vi "fearConditioningOld.vi"() -> ()   [LabVIEW 2010]
uses:
  <vilib>/DAQmx/write.llb/DAQmx Write (Digital Bool 1Line 1Point).vi
  GlobalFear.vi
  <vilib>/daqmx/miscellaneous.llb/DAQmx Fill In Error Info.vi
  <vilib>/measure/NI_MABase.lvlib
panel:
  in  "Pre CS\ntime":dbl=50.0
  in  "stop 2":bool
  in  "stop":bool
  out "Start":bool
  in  "Start":bool
  out "Copleted":bool
  in  "Frequency":dbl=10000.0
  out "Started":bool
  out "Counter":dbl
  in  "ITI":dbl=180.0
  in  "# repeats":dbl=10.0
  out "Shock":bool
  out "Elapsed  Time":dbl format="%#_3g"
  in  "Shock\nDelay":dbl=-1.0
  in  "Shock \nDuration":dbl=-1.0
  in  "Audio \nDuration":dbl=30.0
  out "Audio":bool
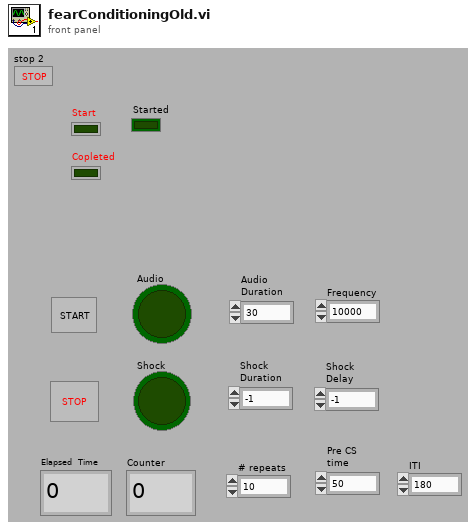
[diagram p1: front panel]
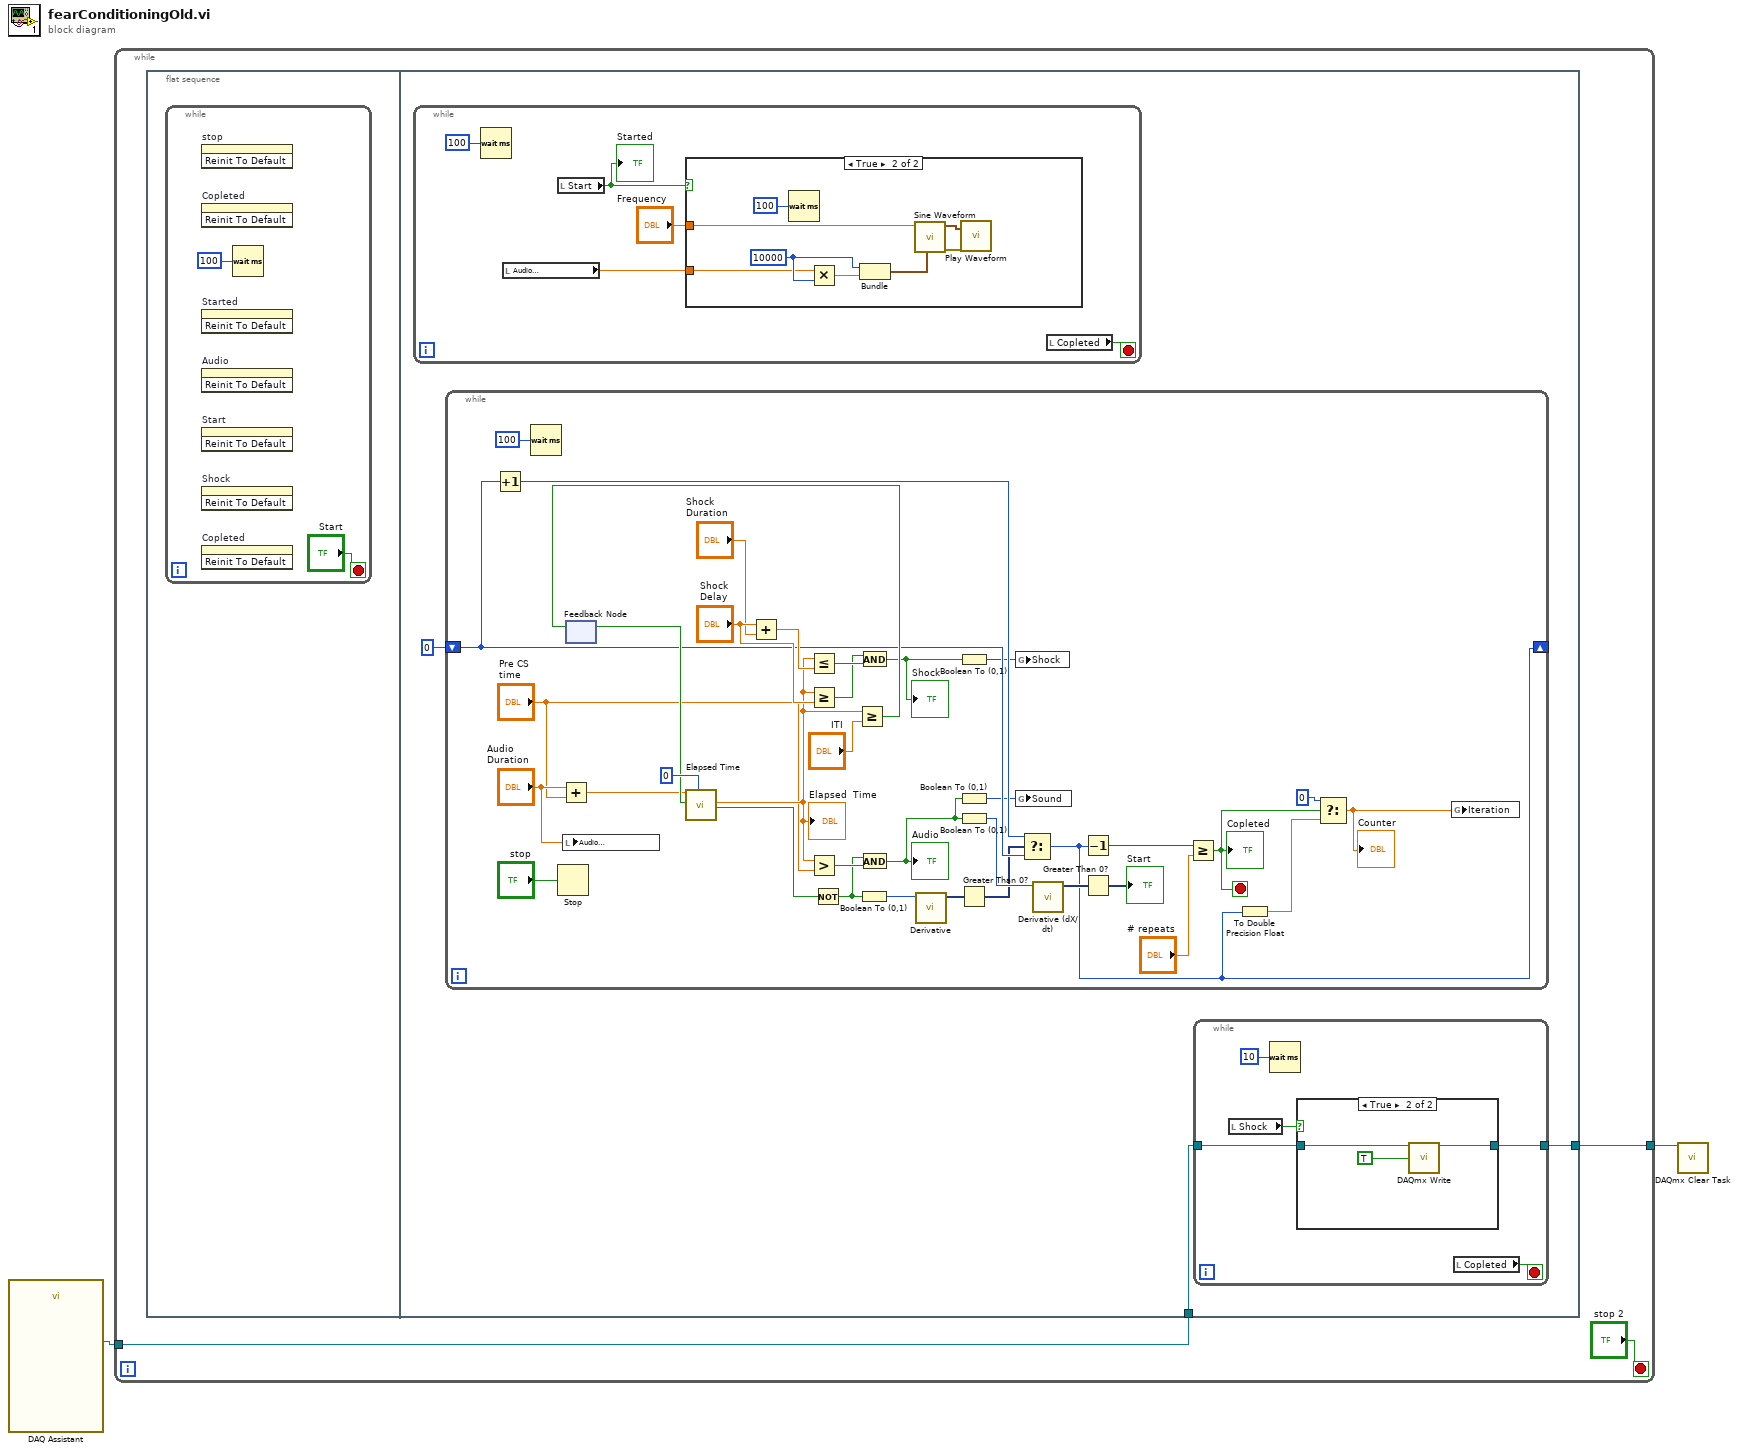
[diagram p0: block diagram]
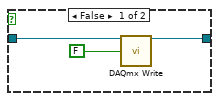
[diagram p2: hidden frame]
diagram:
  n1 = call "DAQ Assistant"() -> ("task out"=w2:refnum<k21>)  [unwired: 18 in, 1 out]
  n2 = while {
    tunnel: w2 -> [w4]
    tunnel: [w3] -> w1
    stop <- "stop 2" stop-if-true
    n3 = flat-sequence {
      tunnel: w4 -> [w9]
      tunnel: [w8] -> w3
      frame #0 {
        n4 = while {
          stop <- "Start" stop-if-true
          n5 = invoke on="stop" class="Bool" method="Reinit To Default"() -> ()  [unwired: 3 in, 3 out]
          n6 = invoke on="Copleted" class="Bool (strict)" method="Reinit To Default"() -> ()  [unwired: 3 in, 3 out]
          n7 = invoke on="Started" class="Bool (strict)" method="Reinit To Default"() -> ()  [unwired: 3 in, 3 out]
          n8 = invoke on="Audio" class="Bool (strict)" method="Reinit To Default"() -> ()  [unwired: 3 in, 3 out]
          n9 = invoke on="Start" class="Bool (strict)" method="Reinit To Default"() -> ()  [unwired: 3 in, 3 out]
          n10 = invoke on="Shock" class="Bool (strict)" method="Reinit To Default"() -> ()  [unwired: 3 in, 3 out]
          n11 = invoke on="Copleted" class="Bool (strict)" method="Reinit To Default"() -> ()  [unwired: 3 in, 3 out]
          n12 = Wait (ms)(milliseconds to wait=100) -> ()  [unwired: 1 out]
        }
      }
      frame #1 {
        n13 = while {
          stop <- w62 stop-if-true
          n14 = Wait (ms)(milliseconds to wait=100) -> ()  [unwired: 1 out]
          n15 = local read "Audio \nDuration"() -> (w60:dbl)
          n16 = local read "Start"() -> (w59:bool)
          "Started" <- w59
          n17 = case shown="True" w59 {
            tunnel: "Frequency" -> [_ w67]
            tunnel: w60 -> [_ w66]
            frame False {
            }
            frame True {
              w71 = 10000
              n18 = Wait (ms)(milliseconds to wait=100) -> ()  [unwired: 1 out]
              n19 = Multiply(x=w66, y=w71) -> (x*y=w70:dbl)
              n20 = Bundle(w71, w70) -> (w69:cluster{i32, dbl})  [unwired: 1 in]
              n21 = call <vilib>:"Sine Waveform.vi"("sampling info"=w69, "frequency"=w67) -> ("error out"=w64:errorcluster, "signal out"=w68:waveform(dbl))  [unwired: 8 in]
              n22 = call "Play Waveform"("Data"=w68, "error in"=w64) -> ()  [unwired: 17 in, 1 out]
            }
          }
          n23 = local read "Copleted"() -> (w62:bool)
        }
        n24 = while {
          shift-right: [w23] -> _
          shift-left: 0 -> [w41]
          stop <- w26 stop-if-true
          n25 = Increment(x=w41) -> (x+1=w42:i32)
          n26 = Wait (ms)(milliseconds to wait=100) -> ()  [unwired: 1 out]
          n27 = Stop(stop? (T)="stop") -> ()
          n28 = Add(x="Audio \nDuration", y="Pre CS\ntime") -> (x+y=w36:dbl)
          n29 = local write "Audio \nDuration"("Audio \nDuration") -> ()
          n30 = feedback #1() -> (w48:bool)  [unwired: 1 in]
          n31 = call "Elapsed Time"("Time Target (s)"=w36, "Reset"=w48, "Set Start Time (s)"=0) -> ("Elapsed Time (s)"=w33:dbl, "Time has Elapsed"=w49:bool)  [unwired: 9 in, 6 out]
          "Elapsed  Time" <- w33
          n32 = Add(x="Shock\nDelay", y="Shock \nDuration") -> (x+y=w52:dbl)
          n33 = Less Or Equal?(x=w33, y=w52) -> (x <= y?=w53:bool)
          n34 = Greater Or Equal?(x=w33, y="Shock\nDelay") -> (x >= y?=w51:bool)
          n35 = Greater?(x=w33, y="Pre CS\ntime") -> (0:w34:bool)
          n36 = Not(x=w49) -> (.not. x?=w29:bool)
          n37 = Greater Or Equal?(x=w33, y="ITI") -> (x >= y?=w43:bool)
          n38 = feedback-in #1(w43) -> ()
          n39 = Boolean To (0,1)(Boolean=w29) -> (0, 1=w31:i16)
          n40 = And(x=w51, y=w53) -> (x .and. y?=w39:bool)
          "Shock" <- w39
          n41 = And(x=w29, y=w34) -> (x .and. y?=w35:bool)
          "Audio" <- w35
          n42 = call "Derivative"("Signals"=w31) -> ("Result"=w30:dynamicdata)  [unwired: 5 in, 1 out]
          n43 = Boolean To (0,1)(Boolean=w39) -> (0, 1=w40:i16)
          n44 = Boolean To (0,1)(Boolean=w35) -> (0, 1=w38:i16)
          n45 = Boolean To (0,1)(Boolean=w35) -> (0, 1=w47:i16)
          n46 = Greater Than 0?(x=w30) -> (x > 0?=w28:dynamicdata)
          n47 = global write "GlobalFear.vi" "Shock"(w40) -> ()
          n48 = global write "GlobalFear.vi" "Sound"(w38) -> ()
          n49 = Select(t=w42, s=w28, f=w41) -> (s? t:f=w23:i32)
          n50 = call "Derivative (dX/dt)"("Signals"=w47) -> ("Result"=w46:dynamicdata)  [unwired: 5 in, 1 out]
          n51 = Decrement(x=w23) -> (x-1=w22:i32)
          n52 = Greater Than 0?(x=w46) -> (x > 0?=→"Start":dynamicdata)
          n53 = Greater Or Equal?(x=w22, y="# repeats") -> (x >= y?=w26:bool)
          "Copleted" <- w26
          n54 = To Double Precision Float(number=w23) -> (double precision float=w27:dbl)
          n55 = Select(t=0, s=w26, f=w27) -> (s? t:f=w24:dbl)
          "Counter" <- w24
          n56 = global write "GlobalFear.vi" "Iteration"(w24) -> ()
        }
        n57 = while {
          tunnel: w9 -> [w15]
          tunnel: [w14] -> w8
          stop <- w13 stop-if-true
          n58 = local read "Shock"() -> (w12:bool)
          n59 = Wait (ms)(milliseconds to wait=10) -> ()  [unwired: 1 out]
          n60 = case shown="True" w12 {
            tunnel: w15 -> [w17 w21]
            tunnel: [w16 w19] -> w14
            frame False {
              n61 = call-poly <vilib>:"DAQmx Write.vi"("task/channels in"=w17, "data"=FALSE) -> ("task out"=w16:refnum<k21>)  [unwired: 11 in, 2 out]
            }
            frame True {
              n62 = call-poly <vilib>:"DAQmx Write.vi"("task/channels in"=w21, "data"=TRUE) -> ("task out"=w19:refnum<k21>)  [unwired: 11 in, 2 out]
            }
          }
          n63 = local read "Copleted"() -> (w13:bool)
        }
      }
    }
  }
  n64 = call <vilib>:"DAQmx Clear Task.vi"("task in"=w1) -> ()  [unwired: 14 in, 1 out]
